vi "char_binread.vi"(8 "error in":errorcluster caption="エラー入力（エラーなし）", 9 "byte order":T1(ring)=enum."little-endian", 10 "offset":i64, 11 "ref in":refnum<file>) -> (0 "error out":errorcluster caption="エラー出力", 2 "float":sgl, 3 "ref out":refnum<file>)   [LabVIEW 2015]
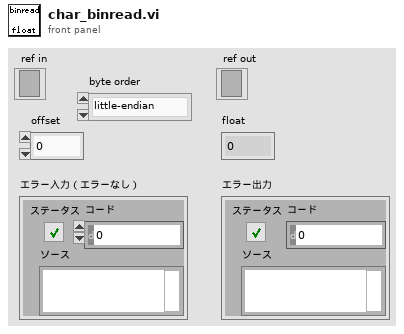
[diagram p1: front panel]
types:
  T1 = enum16{"big-endian, network order", "native, host order", "little-endian"}
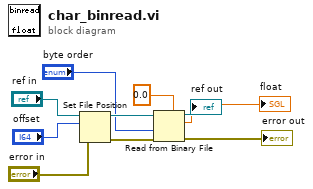
[diagram p0: block diagram]
diagram:
  n1 = Set File Position(offset (in bytes) (0)="offset", refnum="ref in", error in="error in") -> (refnum out=w3:refnum<file>, error out=w4:errorcluster)  [unwired: 1 in]
  n2 = Read from Binary File(5:sgl 0.0, 8:w4, 9:"byte order", 11:w3) -> (0:→"error out":errorcluster, 2:→"float":sgl, 3:→"ref out":refnum<file>)  [unwired: 2 in, 1 out]
